vi "Part 1.vi"(11 "Input":string) -> (3 "Output":i64)   [LabVIEW 2021]
uses:
  32bc949a-07aa-42b8-a6cb-8b275bd12b72.vi
  <userlib>/_OpenG.lib/string/string.llb/Convert EOLs (String)__ogtk.vi
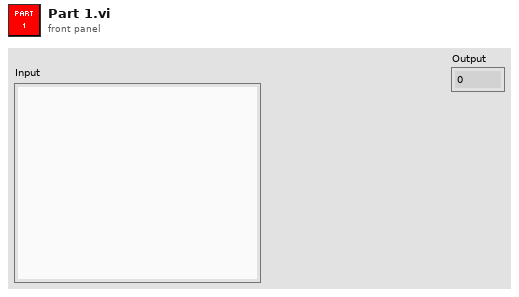
[diagram p1: front panel]
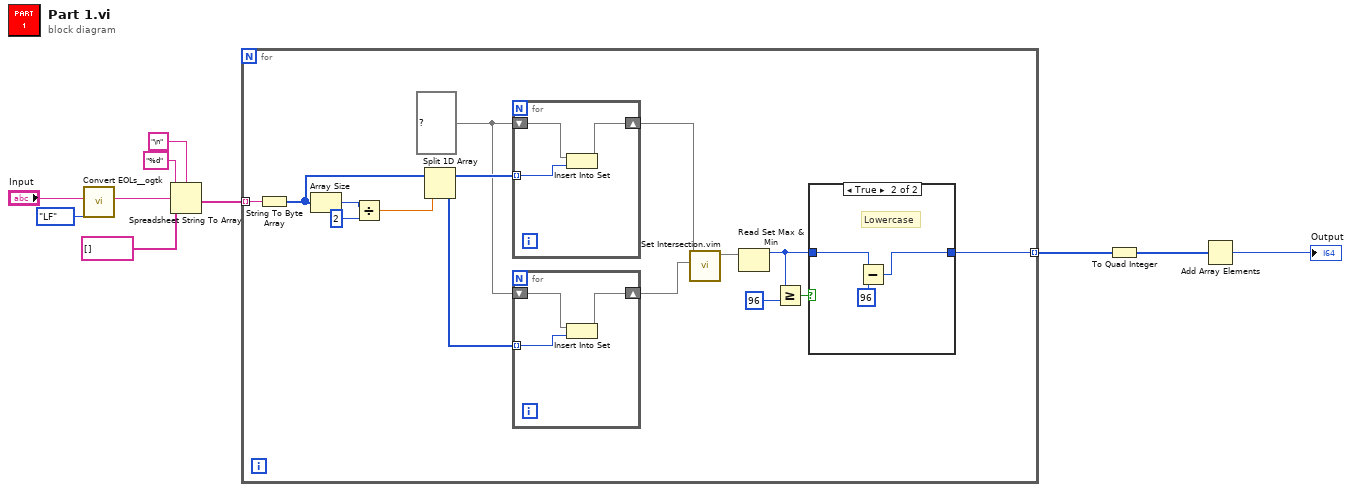
[diagram p0: block diagram]
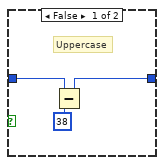
[diagram p2: hidden frame]
diagram:
  n1 = call-poly <userlib>:"Convert EOLs__ogtk.vi"("Convert to:"=enum16{"CR", "LF", "CRLF"}."LF", "String in"="Input") -> ("String out"=w2:string)  [unwired: 9 in]
  n2 = Spreadsheet String To Array(delimiter (Tab)="\n", format string="%d", spreadsheet string=w2, array type (2D Dbl)=string[] []) -> (array=w6:string[])
  n3 = for {
    tunnel: w6 -> [w25] mode=indexing
    tunnel: [w11] -> w5 mode=indexing
    w19 = set{u8} {} ("set in")
    n4 = String To Byte Array(string=w25) -> (unsigned byte array=w21:u8[])
    n5 = Array Size(array=w21) -> (size(s)=w24:i32)
    n6 = Divide(x=w24, y=2) -> (x/y=w22:dbl)
    n7 = Split 1D Array(array=w21, index=w22) -> (first subarray=w20:u8[], second subarray=w18:u8[])
    n8 = for {
      tunnel: w20 -> [w37] mode=indexing
      shift-right: [w35] -> w17
      shift-left: w19 -> [w36]
      n9 = Insert Into Set(10:w37, 11:w36) -> (3:w35:set{u8})  [unwired: 1 out]
    }
    n10 = for {
      tunnel: w18 -> [w34] mode=indexing
      shift-right: [w32] -> w16
      shift-left: w19 -> [w33]
      n11 = Insert Into Set(10:w34, 11:w33) -> (3:w32:set{u8})  [unwired: 1 out]
    }
    n12 = call "Set Intersection.vim"("set 2"=w16, "set 1"=w17) -> ("intersection"=w15:set{u8})  [unwired: 9 in]
    n13 = Read Set Max & Min(11:w15) -> (3:w12:u8)  [unwired: 1 out]
    n14 = Greater Or Equal?(x=w12, y=u8 96) -> (x >= y?=w14:bool)
    n15 = case shown="True" w14 {
      tunnel: w12 -> [w27 w29]
      tunnel: [w26 w30] -> w11
      frame False {
        # "Uppercase"
        n16 = Subtract(x=w27, y=u8 38) -> (x-y=w26:u8)
      }
      frame True {
        # "Lowercase"
        n17 = Subtract(x=w29, y=u8 96) -> (x-y=w30:u8)
      }
    }
  }
  n18 = To Quad Integer(1:w5) -> (0:w3:i64[])
  n19 = Add Array Elements(numeric array=w3) -> (sum=→"Output":i64)
